vi "Create Linear Vector.vi"   [LabVIEW 2017]
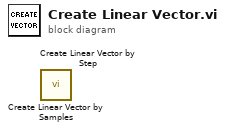
[diagram p0: block diagram]
diagram:
  n1 = call "Create Linear Vector by Samples.vi"() -> ()  [unwired: 9 in, 3 out]
  n2 = call "Create Linear Vector by Step.vi"() -> ()  [unwired: 9 in, 3 out]
